vi "rethinkdb_vi_tree.vi"   [LabVIEW 2017]
uses:
  rethinkdb/RethinkDB.lvclass
  rethinkdb/rethinkdb.lvlib
panel:
  # "SEE DIAGRAM\nFOR VI Tree"
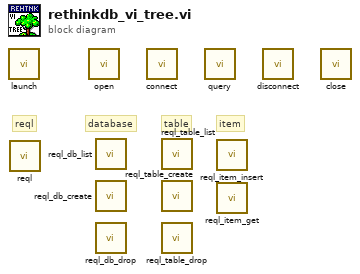
[diagram p0: block diagram]
diagram:
  # "item"
  # "reql"
  # "table"
  # "database"
  n1 = call "launch.vi"() -> ()  [unwired: 11 in, 1 out]
  n2 = call-poly "reql.vi"() -> ()  [unwired: 8 in, 4 out]
  n3 = call "open.vi"() -> ()  [unwired: 10 in, 2 out]
  n4 = call "reql_db_list.vi"() -> ()  [unwired: 8 in, 4 out]
  n5 = call "reql_db_create.vi"() -> ()  [unwired: 8 in, 4 out]
  n6 = call "reql_db_drop.vi"() -> ()  [unwired: 8 in, 4 out]
  n7 = call "connect.vi"() -> ()  [unwired: 10 in, 2 out]
  n8 = call "reql_table_list.vi"() -> ()  [unwired: 8 in, 4 out]
  n9 = call "reql_table_create.vi"() -> ()  [unwired: 8 in, 4 out]
  n10 = call "reql_table_drop.vi"() -> ()  [unwired: 8 in, 4 out]
  n11 = call "query.vi"() -> ()  [unwired: 8 in, 4 out]
  n12 = call "reql_item_insert.vi"() -> ()  [unwired: 8 in, 4 out]
  n13 = call "reql_item_get.vi"() -> ()  [unwired: 8 in, 4 out]
  n14 = call "disconnect.vi"() -> ()  [unwired: 10 in, 2 out]
  n15 = call "close.vi"() -> ()  [unwired: 11 in, 1 out]
